vi "_Start.vi"(6 "EventLogging":refnum<class "EventLoggingService.lvclass">, 8 "error in (no error)":errorcluster, 11 "Loop Data In":T1) -> (0 "error out":errorcluster, 3 "Loop Data":T1)   [LabVIEW 2020, in "Vecto.lvlib" / "RemoteDataService.lvclass"]
uses:
  RemoteDataService.lvclass
  Loop Data.ctl
  SequenceCountService/SequenceCountService.lvclass
  ChannelService/ChannelService.lvclass
  IP Resolver/IP Resolver.lvclass
  Published Group.ctl
  Packet.ctl
  lv-protoc/LV-Proto/Message/Message.lvclass
  Group Data Type.ctl
  Subscription.ctl
  Subscription Info.ctl
  SubscribedDataHandler/SubscribedDataHandler.lvclass
  VectoConfig/Telemetry Config.ctl
  VectoConfig/Telemetry Routing.ctl
  VectoConfig/Endpoint.ctl
  EventLoggingService/EventLoggingService.lvclass
  Event Level.ctl
  EventLoggingService/EventLoggingService.lvclass/EventLoggingService.ctl
  <vilib>/Utility/error.llb/Error Cluster From Error Code.vi
  EventLogHandler/EventLogHandler.lvclass
  Vecto.lvlib
  VectoConfig/VectoConfig.lvlib
panel:
  out "Bound IP":string
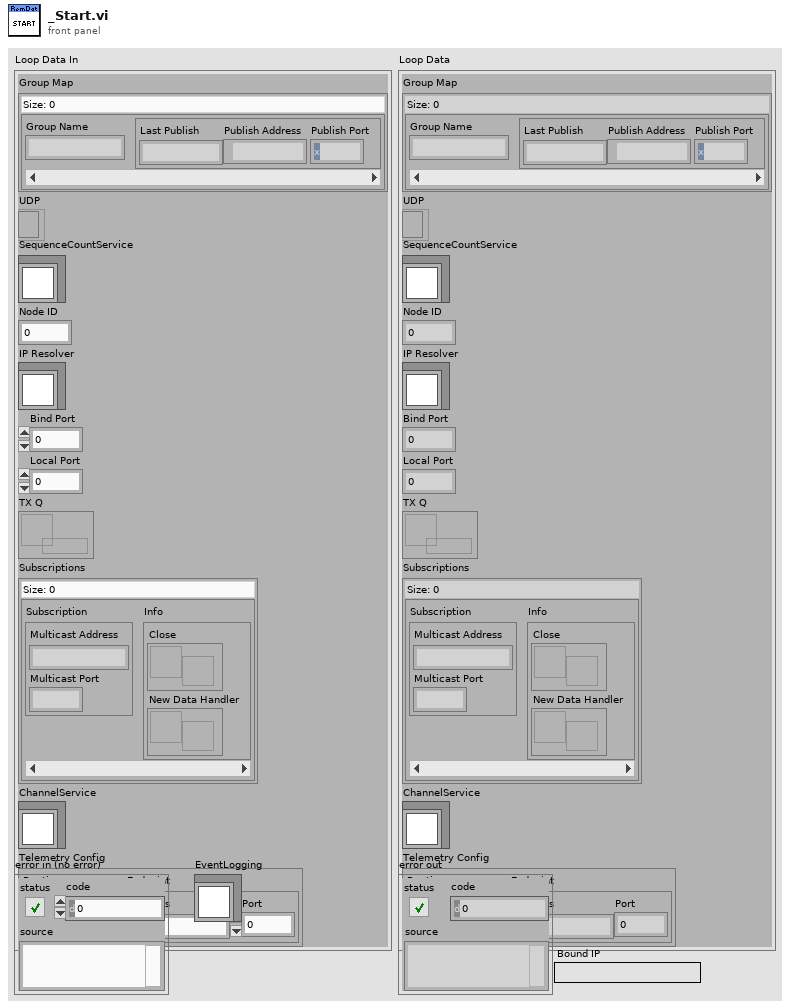
[diagram p1: front panel]
types:
  T1 = typedef "Vecto.lvlib/RemoteDataService.lvclass/Loop Data.ctl" = cluster{"Group Map":map{string, T2}, "UDP":refnum<k16>, "SequenceCountService":refnum<class "SequenceCountService.lvclass">, "Node ID":u32, "IP Resolver":refnum<class "IP Resolver.lvclass">, "Bind Port":u16, "Local Port":u16, "TX Q":refnum<queue>, "Subscriptions":map{T3, T4}, "ChannelService":refnum<class "ChannelService.lvclass">, "Telemetry Config":T5}
  T2 = typedef "Vecto.lvlib/RemoteDataService.lvclass/Published Group.ctl" = cluster{"Last Publish":dbl, "Publish Address":u32, "Publish Port":u16}
  T3 = typedef "Vecto.lvlib/RemoteDataService.lvclass/Subscription.ctl" = cluster{"Multicast Address":string, "Multicast Port":u16}
  T4 = typedef "Vecto.lvlib/RemoteDataService.lvclass/Subscription Info.ctl" = cluster{"Close":refnum<user-event>, "New Data Handler":refnum<user-event>}
  T5 = typedef "VectoConfig.lvlib/Telemetry Config.ctl" = cluster{"Routing":T6, "Endpoint":T7}
  T6 = typedef "VectoConfig.lvlib/Telemetry Routing.ctl" = enum16{"Multicast", "Unicast"}
  T7 = typedef "VectoConfig.lvlib/Endpoint.ctl" = cluster{"Address":string, "Port":u16}
  T8 = typedef "Vecto.lvlib/Event Level.ctl" = enum16{"Debug", "Info", "Warning", "Error"}
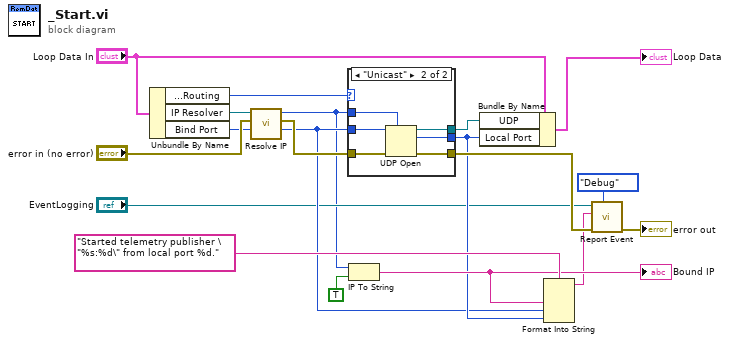
[diagram p0: block diagram]
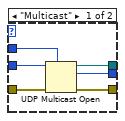
[diagram p2: hidden frame]
diagram:
  n1 = Unbundle By Name("Loop Data In") -> ("Telemetry Config.Routing"=w2:T6, "IP Resolver"=w3:refnum<class "IP Resolver.lvclass">, "Bind Port"=w8:u16)
  n2 = call "Resolve IP.vi"("error in (no error)"="error in (no error)", "IP Resolver in"=w3) -> ("error out"=w17:errorcluster, "U32 Address"=w1:u32)  [unwired: 8 in]
  n3 = case shown="\"Unicast\"" w2 {
    tunnel: [w24 w29] -> w16
    tunnel: [w23 w27] -> w14
    tunnel: w17 -> [w22 w30]
    tunnel: [w21 w28] -> w9
    tunnel: w8 -> [w20 w25]
    tunnel: w1 -> [w19 w26]
    frame "Multicast" {
      n4 = UDP Multicast Open(7:w19, 8:w22, 11:w20) -> (0:w24:errorcluster, 2:w21:u16, 3:w23:refnum<k16>)  [unwired: 1 in, 1 out]
    }
    frame "Unicast" {
      n5 = UDP Open(7:w26, 8:w30, 11:w25) -> (port=w27:refnum<k16>, 0:w29:errorcluster, 2:w28:u16)  [unwired: 2 in]
    }
  }
  n6 = IP To String(1:TRUE ("dot notation? (F)"), 2:w1) -> (0:w10:string)
  "Bound IP" <- w10
  n7 = Bundle By Name(cluster="Loop Data In", "UDP"=w14, "Local Port"=w9) -> (→"Loop Data":T1)
  n8 = Format Into String(format string="Started telemetry publisher \"%s:%d\" from local port %d.", w10, w8, w9) -> (resulting string=w6:string)  [unwired: 2 in, 1 out]
  n9 = call "Report Event.vi"("Event Level (Info)"=Event_Level."Debug", "error in (no error)"=w16, "Message"=w6, "EventLoggingService in"="EventLogging") -> ("error out"=→"error out":errorcluster)  [unwired: 6 in, 1 out]
